vi "Open Implementations.vi"(0 "Class in":refnum<vi>, 1 "Implementation List":string[](array[string]), 2 "Method Name":string, 3 "error in (no error)":errorcluster, 4 "Activate BD":bool) -> (5 "Class out":refnum<vi>, 6 "error out":errorcluster)   [LabVIEW 2020, in "Choose Implementation Dialog.lvlib"]
uses:
  Choose Implementation Dialog.lvlib
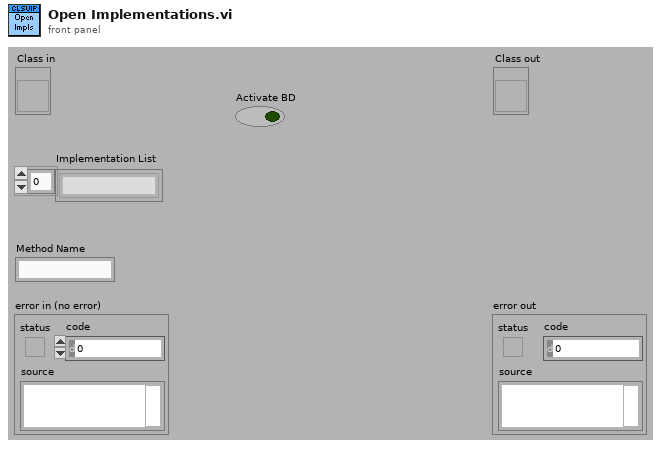
[diagram p1: front panel]
types:
  T1 = enum32{"Invalid", "Standard", "Closed", "Hidden", "Minimized", "Maximized"}
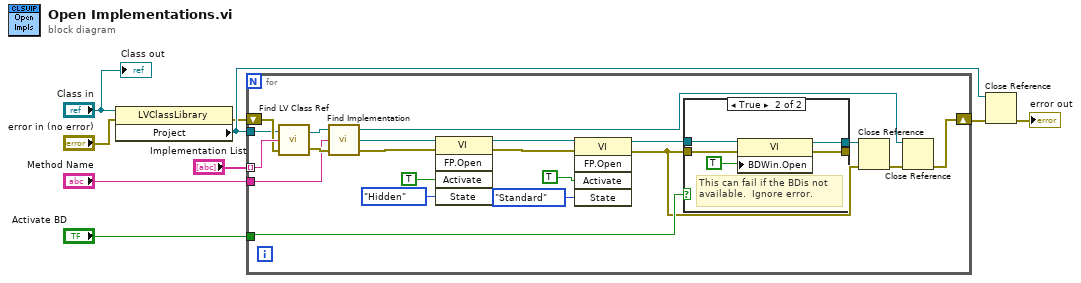
[diagram p0: block diagram]
diagram:
  n1 = property class="LVClassLibrary"(reference="Class in", error in="error in (no error)") -> (error out=w8:errorcluster, "Project"=w9:refnum<vi>)  [unwired: 1 out]
  n2 = for {
    tunnel: "Implementation List" -> [w30] mode=indexing
    tunnel: "Method Name" -> [w27]
    tunnel: "Activate BD" -> [w25]
    shift-right: [w22] -> w5
    shift-left: w8 -> [w23]
    tunnel: w9 -> [w19]
    n3 = call "Find LV Class Ref.vi"("error in (no error)"=w23, "Item ID"=w30, "Expected Project"=w19) -> ("error out"=w28:errorcluster, "LVClassLibrary Refnum"=w29:refnum<vi>)
    n4 = call "Find Implementation.vi"("error in"=w28, "Method Name"=w27, "Class in"=w29) -> ("error out"=w14:errorcluster, "VI"=w15:refnum<vi>, "Class out"=w20:refnum<vi>)
    n5 = invoke class="VI" method="FP.Open"(reference=w15, error in=w14, "Activate"=TRUE ("Activate?"), "State"=T1."Hidden") -> (reference out=w12:refnum<vi>, error out=w13:errorcluster)  [unwired: 1 in, 3 out]
    n6 = invoke class="VI" method="FP.Open"(reference=w12, error in=w13, "Activate"=TRUE ("Activate?"), "State"=T1."Standard") -> (reference out=w26:refnum<vi>, error out=w17:errorcluster)  [unwired: 1 in, 3 out]
    n7 = case shown="True" w25 {
      tunnel: w26 -> [w31 w37]
      tunnel: w17 -> [w32 w36]
      tunnel: [w31 w34] -> w24
      tunnel: [w32 w33] -> _
      frame False {
      }
      frame True {
        # "This can fail if the BDis not \navailable.  Ignore error."
        n8 = property class="VI"(reference=w37, error in=w36, "BDWin.Open"=TRUE ("Block Diagram Window:Open")) -> (reference out=w34:refnum<vi>, error out=w33:errorcluster)
      }
    }
    n9 = Close Reference(reference=w24, error in (no error)=w17) -> (error out=w21:errorcluster)
    n10 = Close Reference(reference=w20, error in (no error)=w21) -> (error out=w22:errorcluster)
  }
  n11 = Close Reference(reference=w9, error in (no error)=w5) -> (error out=→"error out":errorcluster)
  "Class out" <- "Class in"
